vi "init_34401A.vi"(8 "Rozsah 34401A":enum16{"10 mA", "100 mA", "1 A", "3 A"}(ring), 9 "Rozliseni 34401A":T1(ring)) -> (2 "Command String":string)   [LabVIEW 2021]
panel:
  # "34401A - AMPERMET"
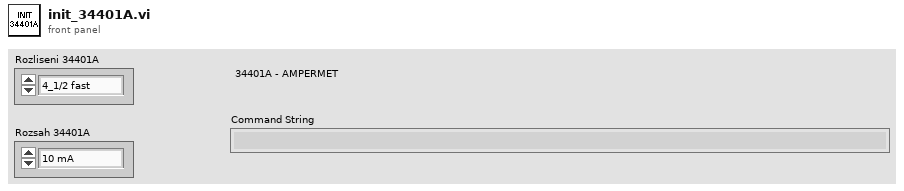
[diagram p1: front panel]
types:
  T1 = enum16{"4_1/2 fast", "4_1/2 slow", "5_1/2 fast", "5_1/2 slow", "6_1/2 fast", "6_1/2 slow"}
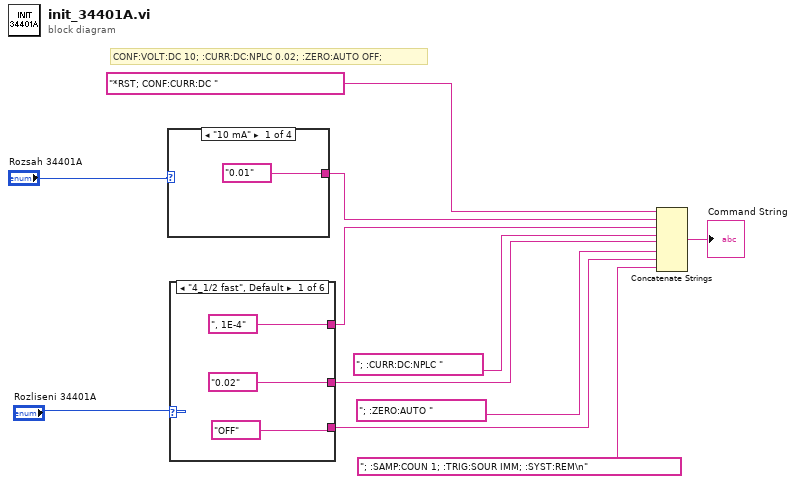
[diagram p0: block diagram]
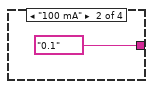
[diagram p2: hidden frame]
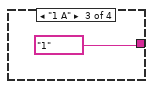
[diagram p3: hidden frame]
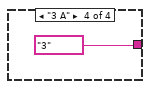
[diagram p4: hidden frame]
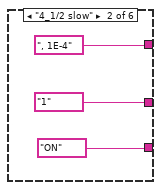
[diagram p5: hidden frame]
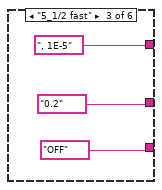
[diagram p6: hidden frame]
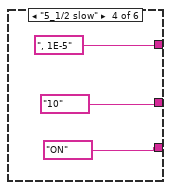
[diagram p7: hidden frame]
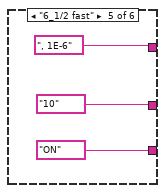
[diagram p8: hidden frame]
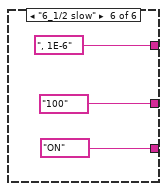
[diagram p9: hidden frame]
diagram:
  # "CONF:VOLT:DC 10; :CURR:DC:NPLC 0.02; :ZERO:AUTO OFF;"
  n1 = case shown="\"10 mA\"" "Rozsah 34401A" {
    tunnel: ["0.01" "0.1" "1" "3"] -> w9
    frame "10 mA" {
    }
    frame "100 mA" {
    }
    frame "1 A" {
    }
    frame "3 A" {
    }
  }
  n2 = case shown="\"4_1/2 fast\", Default" "Rozliseni 34401A" {
    tunnel: ["0.02" "1" "0.2" "10" "10" "100"] -> w6
    tunnel: ["OFF" "ON" "OFF" "ON" "ON" "ON"] -> w5
    tunnel: [", 1E-4" ", 1E-4" ", 1E-5" ", 1E-5" ", 1E-6" ", 1E-6"] -> w8
    frame "4_1/2 fast", Default {
    }
    frame "4_1/2 slow" {
    }
    frame "5_1/2 fast" {
    }
    frame "5_1/2 slow" {
    }
    frame "6_1/2 fast" {
    }
    frame "6_1/2 slow" {
    }
  }
  n3 = Concatenate Strings("*RST; CONF:CURR:DC ", w9, w8, "; :CURR:DC:NPLC ", w6, "; :ZERO:AUTO ", w5, "; :SAMP:COUN 1; :TRIG:SOUR IMM; :SYST:REM\n") -> (→"Command String":string)
